vi "State_Machine.vi"(8 "error in (no error)":errorcluster caption="entrée d'erreur (pas d'erreur)", 11 "Get_Voltage en entrée":refnum<class "Nodon_Check_ZCR_Calibration.lvclass">) -> (0 "error out":errorcluster caption="sortie d'erreur", 2 "Json_String":string, 3 "Get_Voltage en sortie":refnum<class "Nodon_Check_ZCR_Calibration.lvclass">)   [LabVIEW 2020, in "Library Test.lvlib" / "Nodon_Check_ZCR_Calibration.lvclass"]
uses:
  Nodon_Check_ZCR_Calibration.lvclass
  C:/Users/ngarcin/OneDrive - Altyor/Standard TB/Suite TB45/Class/Test/Test (Default)/Test (Default).lvclass
  Commun VI/TypeDef/Variable Printable.ctl
  Test_Without_Instr/Test_Without_Inst.lvclass
  Commun VI/Library Commun.lvlib
  Commun VI/Nodon_ZCR/Nodon_ZCR.lvclass
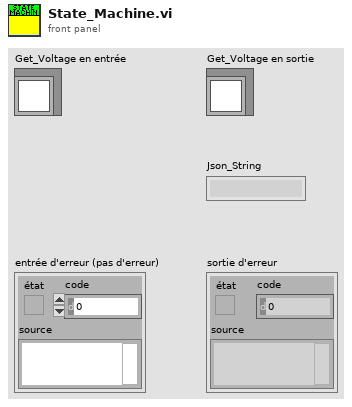
[diagram p1: front panel]
types:
  T1 = typedef "Variable Printable.ctl" = string
  T2 = enum16{"Get Variable", "Get All Variables", "Set Variable", "Delete Variable", "Delete All Variable"}
  T3 = cluster{"Décallage sinus On":dbl, "Décallage sinus Off":dbl}
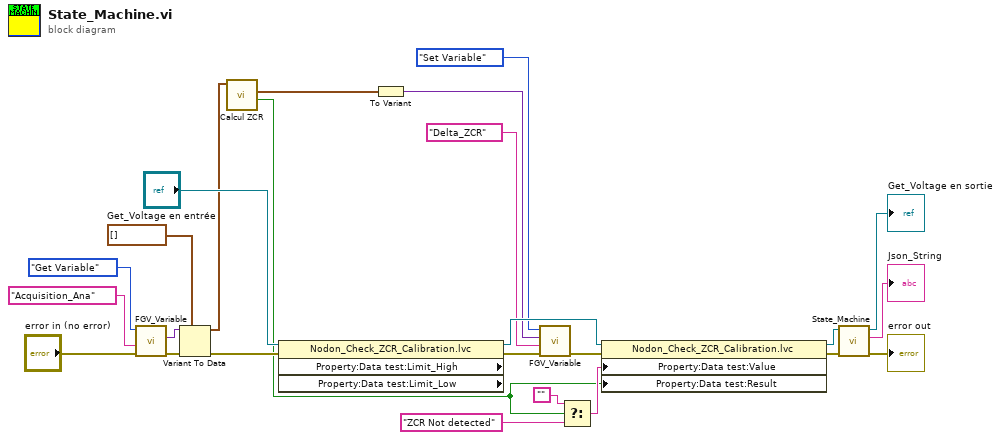
[diagram p0: block diagram]
diagram:
  n1 = call "FGV_Variable.vi"("error in (no error)"="error in (no error)", "Variable"=T1 "Acquisition_Ana", "Function"=T2."Get Variable") -> ("error out"=w20:errorcluster, "Data Out"=w19:variant)  [unwired: 6 in, 1 out]
  n2 = Variant To Data(error in=w20, type=waveform(dbl)[] [] ("data"), Variant=w19) -> (data=w11:waveform(dbl)[], error out=w14:errorcluster)
  n3 = call "Calcul ZCR.vi"("ZCR Signal Input"=w11) -> ("ZCR Valid"=w2:bool, "Controle Decalage"=w7:T3)  [unwired: 8 in, 1 out]
  n4 = property class="Nodon_Check_ZCR_Calibration.lvc" props=["Property:Data test:Limit_High", "Property:Data test:Limit_Low"](reference="Get_Voltage en entrée", error in=w14) -> (reference out=w12:refnum<class "Nodon_Check_ZCR_Calibration.lvclass">, error out=w8:errorcluster)  [unwired: 2 out]
  n5 = To Variant(anything=w7) -> (Variant=w6:variant)
  n6 = call "FGV_Variable.vi"("error in (no error)"=w8, "Variable"=T1 "Delta_ZCR", "Data In"=w6, "Function"=T2."Set Variable") -> ("error out"=w1:errorcluster)  [unwired: 5 in, 2 out]
  n7 = Select(t="", s=w2, f="ZCR Not detected" ("cas faux")) -> (s? t:f=w3:string)
  n8 = property class="Nodon_Check_ZCR_Calibration.lvc"(reference=w12, error in=w1, "Property:Data test:Value"=w3, "Property:Data test:Result"=w2) -> (reference out=w15:refnum<class "Nodon_Check_ZCR_Calibration.lvclass">, error out=w16:errorcluster)
  n9 = call-parent "State_Machine.vi"("error in (no error)"=w16, "Test_Without_Inst en entrée"=w15) -> ("error out"=→"error out":errorcluster, "Json_String"=→"Json_String":string, "Test_Without_Inst en sortie"=→"Get_Voltage en sortie":refnum<class "Nodon_Check_ZCR_Calibration.lvclass">)  [unwired: 7 in]
